vi "Dialog.vi"() -> ()   [LabVIEW 2013]
panel:
  in  "No Button":bool
  in  "Yes Button":bool
  out "T/F":bool
  # "Start over tracking?"
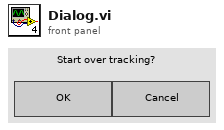
[diagram p1: front panel]
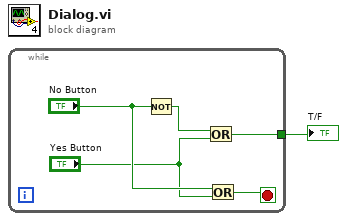
[diagram p0: block diagram]
diagram:
  n1 = while {
    tunnel: [w5] -> w1
    stop <- w4 stop-if-true
    n2 = Not(x="No Button") -> (.not. x?=w6:bool)
    n3 = Or(x=w6, y="Yes Button") -> (x .or. y?=w5:bool)
    n4 = Or(x="No Button", y="Yes Button") -> (x .or. y?=w4:bool)
  }
  "T/F" <- w1
